vi "Create CE measurements for SS.vi"(8 "error in (no error)":errorcluster, 11 "SS measurement":T2 {"PJVS reference voltages array of vector cluster"."PJVS reference voltages vector" format="%#_3p"; "PJVS frequencies (Hz)" format="%#_3p"; "Record lengths (multiples of periods)" format="%#_3p"; "Sampling frequencies (Hz)" format="%#_3p"; "Signal amplitudes (V)" format="%#_3p"; "Signal frequencies (Hz)" format="%#_3p"}) -> (0 "error out":errorcluster, 1 "CE measurement after":T1={"Signal frequencies (Hz) T"=[1000.0], "Signal amplitudes (V) T"=[0.707], "Sampling frequencies (Hz) T"=[10000000.0], "Record lengths (multiples of periods) T"=[10000.0], "TWM data root directory"=path "", "TWM mreasurements directories"=[], "Calculate RMS from samples"=FALSE, "Algorithm to use"="TWM-WFFT", "Quantity to read"="TWM-WFFT", "Settle down after AC source change (s) T"=1.0, "Skip PJVS setup"=FALSE, "Measurement template file"=path "", "Row of START keyword T"=0, "Row of STOP keyword T"=0, "Measurement template line T"=[], "Switch position T"=[10000.0], "FR fit mat file T"=path "", "Recalculate-skip already calculated"=FALSE} {"Switch position T" format="%#_3p"; "Record lengths (multiples of periods) T" format="%#_3p"; "Sampling frequencies (Hz) T" format="%#_3p"; "Signal amplitudes (V) T" format="%#_3p"; "Signal frequencies (Hz) T" format="%#_3p"}, 2 "CE measurement before":T1={"Signal frequencies (Hz) T"=[1000.0], "Signal amplitudes (V) T"=[0.707], "Sampling frequencies (Hz) T"=[10000000.0], "Record lengths (multiples of periods) T"=[10000.0], "TWM data root directory"=path "", "TWM mreasurements directories"=[], "Calculate RMS from samples"=FALSE, "Algorithm to use"="TWM-WFFT", "Quantity to read"="TWM-WFFT", "Settle down after AC source change (s) T"=1.0, "Skip PJVS setup"=FALSE, "Measurement template file"=path "", "Row of START keyword T"=0, "Row of STOP keyword T"=0, "Measurement template line T"=[], "Switch position T"=[10000.0], "FR fit mat file T"=path "", "Recalculate-skip already calculated"=FALSE} {"Switch position T" format="%#_3p"; "Record lengths (multiples of periods) T" format="%#_3p"; "Sampling frequencies (Hz) T" format="%#_3p"; "Signal amplitudes (V) T" format="%#_3p"; "Signal frequencies (Hz) T" format="%#_3p"}, 3 "SS measurement out":T2={"Signal frequencies (Hz)"=[1000.0], "Signal amplitudes (V)"=[0.707], "Sampling frequencies (Hz)"=[10000000.0], "Record lengths (multiples of periods)"=[10000.0], "Calculate results"=FALSE, "Algorithm"="TWM-PJVSSubS", "TWM data directories"=[], "TWM data directories relative"=[], "Settle down after AC source change (s)"=1.0, "PJVS frequencies (Hz)"=[1000.0], "PJVS reference voltages array of vector cluster"=[], "Requested PJVS steps"=[20], "Measure CE"=FALSE, "Measure CE before"=FALSE, "Measure CE after"=FALSE, "Single point CE measurement"=FALSE, "original CE template path"=path "", "new CE template path before SS"=path "", "new CE template path before SS relative"=path "", "new CE template path after SS"=path "", "new CE template path after SS relative"=path "", "original CE fit path"=path "", "new CE fit path before SS"=path "", "new CE fit path before SS relative"=path "", "new CE fit path after SS"=path "", "new CE fit path after SS relative"=path "", "Measure digitizer gain"=FALSE, "Measure digitizer gain before"=FALSE, "Measure digitizer gain after"=FALSE, "Digitizer gain"=0.0, "Data folder"=path "", "FR fit path"=path "", "new FR fit path relative"=path "", "Rs"=0, "Re"=0, "SS measurement info files"=[]} {"PJVS reference voltages array of vector cluster"."PJVS reference voltages vector" format="%#_3p"; "PJVS frequencies (Hz)" format="%#_3p"; "Record lengths (multiples of periods)" format="%#_3p"; "Sampling frequencies (Hz)" format="%#_3p"; "Signal amplitudes (V)" format="%#_3p"; "Signal frequencies (Hz)" format="%#_3p"})   [LabVIEW 2020]
doc: "Prepare CE measurement for SS measurement - proper paths, if needed modify for single point CE mesurement."
uses:
  SS Measurement/Type definitions/SS measurement.ctl
  CE Measurement/Type definitions/CE measurement.ctl
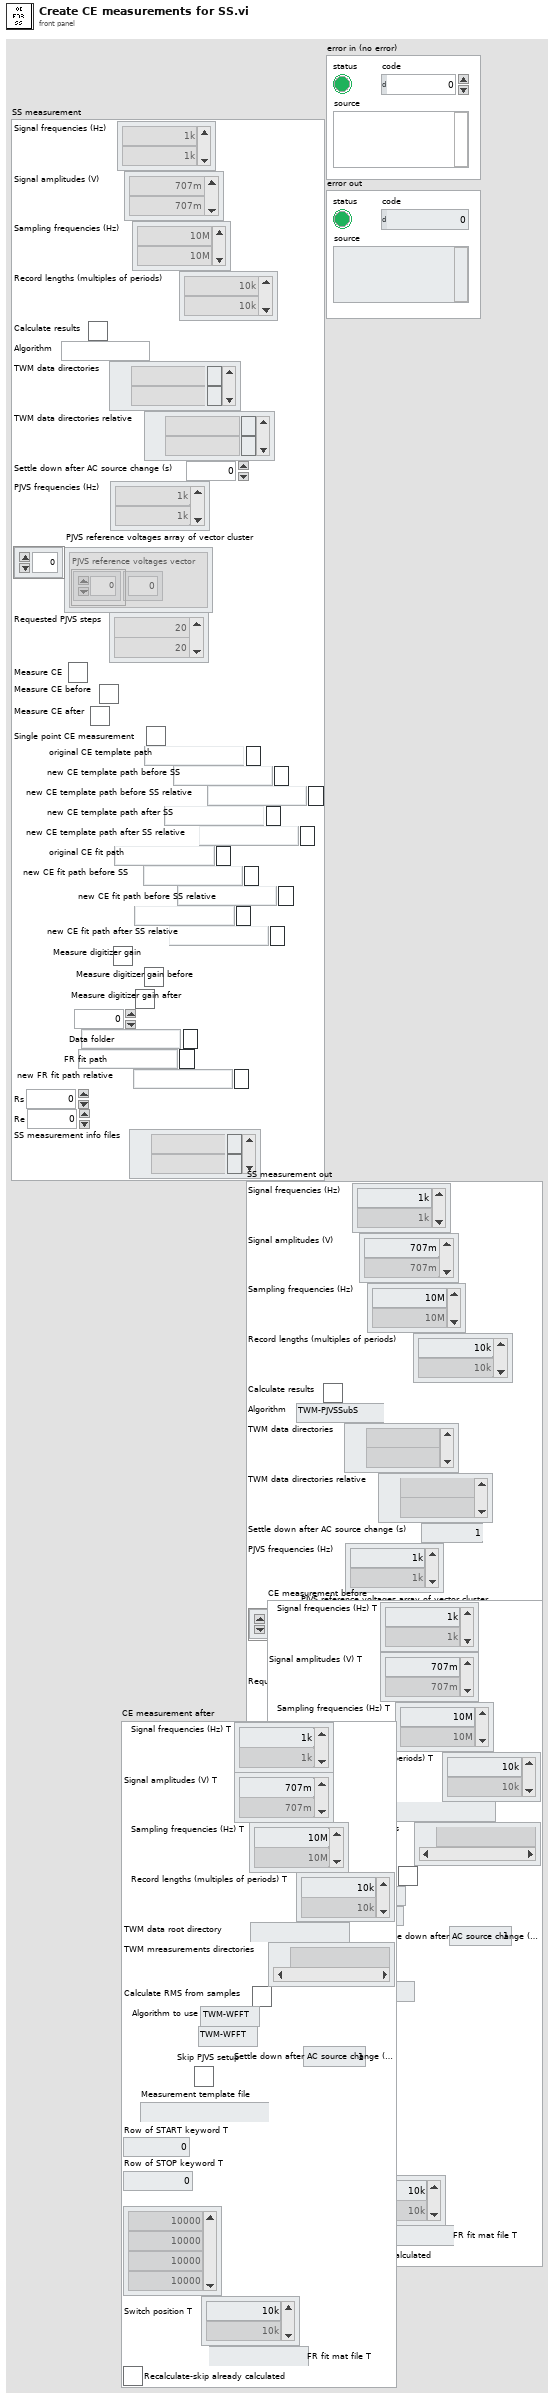
[diagram p1: front panel]
types:
  T1 = typedef "CE measurement.ctl" = cluster{"Signal frequencies (Hz) T":dbl[], "Signal amplitudes (V) T":dbl[], "Sampling frequencies (Hz) T":dbl[], "Record lengths (multiples of periods) T":dbl[], "TWM data root directory":path, "TWM mreasurements directories":path[], "Calculate RMS from samples":bool, "Algorithm to use":string, "Quantity to read":string, "Settle down after AC source change (s) T":dbl, "Skip PJVS setup":bool, "Measurement template file":path, "Row of START keyword T":i32, "Row of STOP keyword T":i32, "Measurement template line T":i32[], "Switch position T":dbl[], "FR fit mat file T":path, "Recalculate-skip already calculated":bool}
  T2 = typedef "SS measurement.ctl" = cluster{"Signal frequencies (Hz)":dbl[], "Signal amplitudes (V)":dbl[], "Sampling frequencies (Hz)":dbl[], "Record lengths (multiples of periods)":dbl[], "Calculate results":bool, "Algorithm":string, "TWM data directories":path[], "TWM data directories relative":path[], "Settle down after AC source change (s)":dbl, "PJVS frequencies (Hz)":dbl[], "PJVS reference voltages array of vector cluster":cluster{"PJVS reference voltages vector":dbl[]}[], "Requested PJVS steps":u32[], "Measure CE":bool, "Measure CE before":bool, "Measure CE after":bool, "Single point CE measurement":bool, "original CE template path":path, "new CE template path before SS":path, "new CE template path before SS relative":path, "new CE template path after SS":path, "new CE template path after SS relative":path, "original CE fit path":path, "new CE fit path before SS":path, "new CE fit path before SS relative":path, "new CE fit path after SS":path, "new CE fit path after SS relative":path, "Measure digitizer gain":bool, "Measure digitizer gain before":bool, "Measure digitizer gain after":bool, "Digitizer gain":dbl, "Data folder":path, "FR fit path":path, "new FR fit path relative":path, "Rs":i32, "Re":i32, "SS measurement info files":path[]}
  T3 = typedef "Type definitions to be saved.ctl" = cluster{"Common properties":T4, "AC Source":T5, "DC meter":T7, "CE measurement":T1, "FR measurement":T9, "FR template":T10, "CE template":T11, "PJVS":T12, "SS measurement":T2, "AC sync source":T5, "DG measurement":T16}
  T4 = typedef "Common properties.ctl" = cluster{"Measurement status ref":refnum<vi>, "TWM Status ref":refnum<vi>, "Abort ref":refnum<vi>, "Skip waiting ref":refnum<vi>, "GNU Octave path":path, "TWM+QWTB path":path, "lvlib path":path, "TWM pipe":string, "PJVS status ref":refnum<vi>, "WAC path":path}
  T5 = typedef "AC Source.ctl" = cluster{"AC Source type":T6, "VISA":refnum<visa-resource-name>, "Ref. clock (Hz)":dbl, "status ref":refnum<vi>, "Fluke 57XX wideband output":bool, "Fluke 57XX ignore errors":bool, "Synchronization by AC signal":bool}
  T6 = typedef "AC Source type.ctl" = enum16{"Fluke 5XXX calibrator", "Tektronix AFG3000 series", "dummy", "Agilent 331xxA to 332xxA", "Agilent 335xxA to 336xxA"}
  T7 = typedef "DC meter.ctl" = cluster{"DC meter type":T8, "DC meter VISA":refnum<visa-resource-name>, "NPLC":dbl, "status ref":refnum<vi>}
  T8 = typedef "DC meter type.ctl" = enum16{"H/A/K 3458", "Fluke 8508A", "dummy", "Keithley 2182"}
  T9 = typedef "FR measuement.ctl" = cluster{"Measurement frequencies (Hz)":dbl[], "Sampling frequency (Hz)":dbl, "Signal amplitude (V)":dbl, "AC-DC settle time (s)":dbl, "Record length (multiples of period)":dbl[], "Measurement template file":path, "Row of START keyword":i32, "Row of STOP keyword":i32, "Calculate RMS from samples":bool, "AC-DC warm up time (s)":dbl, "Measurement template line":i32[], "DC meter readings No.":i32, "Algorithm":string, "Simultaneous measurement":bool, "Recalculate-skip already calculated":bool}
  T10 = typedef "FR template.ctl" = cluster{"Keywords column":i32, "Sig. freq. column":i32, "Rec. len. column":i32, "Meas. points. row min to read":i32, "Meas. points. row max to read":i32, "Properties column":i32, "Properties row start":i32, "Properties row end":i32, "Keyword START regexp":string, "Keyword STOP regexp":string, "HW data column":i32, "HW data row start":i32, "HW data row end":i32, "TIme and date column start":i32, "Digitizer value column start ":i32, "DC mean column start ":i32, "DC readings column start":i32}
  T11 = typedef "CE template.ctl" = cluster{"Keywords column":i32, "Sig. freq. column":i32, "Rec. len. column":i32, "Switch pos column":i32, "Meas. points. row min to read":i32, "Meas. points. row max to read":i32, "Properties column":i32, "Properties row start":i32, "Properties row end":i32, "Keyword START regexp":string, "Keyword STOP regexp":string, "HW data column":i32, "HW data row start":i32, "HW data row end":i32, "TIme and date column start":i32, "Digitizer value column start ":i32}
  T12 = typedef "PJVS.ctl" = cluster{"PJVS type":T13, "Status Refnum":refnum<vi>, "AC-supraVOLTcontrol":cluster{"IP address:port (0.0.0.0:0000)":string, "Timeouts":T14, "Simulation mode":bool, "Debug mode":bool}, "NPL bias source":cluster{"DataSocketCluster":T15}, "Manual PJVS":cluster{"PJVS frequency (Hz)":dbl, "Reference voltages (V)":dbl[], "File with PJVS voltages":path}, "VTT PJVS":cluster{"some VTT only property":string}}
  T13 = typedef "PJVS Type.ctl" = enum16{"AC-supraVOLTcontrol", "JV modified NPL bias control", "Manual PJVS", "VTT PJVS"}
  T14 = typedef "ACSVcontrol-driver.lvlib/Timeouts.ctl" = cluster{"TCP Read & Write (ms)":i32, "Sensors readout":i32, "PJVS setup":i32, "Nullmeter readout":i32, "Multiplexer setup":i32, "57XX setup":i32, "Generator setup":i32, "Synthesizer setup":i32, "Sampler readout":i32}
  T15 = typedef "DataSocketCluster external.ctl" = cluster{"Server Machine":string, "Client Machine":string, "Data":string, "TimeStamp":dbl, "Count":i32, "Target Process":string}
  T16 = typedef "DG measurement.ctl" = cluster{"Sampling frequencies (Hz)":dbl[], "Requested PJVS frequencies (Hz)":dbl[], "Requested PJVS waveform amplitudes (V)":dbl[], "Record lengths (multiples of PJVS periods)":dbl[], "Requested PJVS steps":u32[], "Switch position":dbl, "Settle down after PJVS change (s)":dbl, "Rs":i32, "Re":i32, "Algorithm":string, "Calculate results":bool, "Data folder":path, "TWM data directories":path[], "TWM data directories relative":path[], "DG measurement info files":path[], "Set PJVS frequencies (Hz)":dbl[], "Set PJVS reference voltages array of vector cluster":cluster{"PJVS reference voltages vector":dbl[]}[], "Set PJVS steps":u32[]}
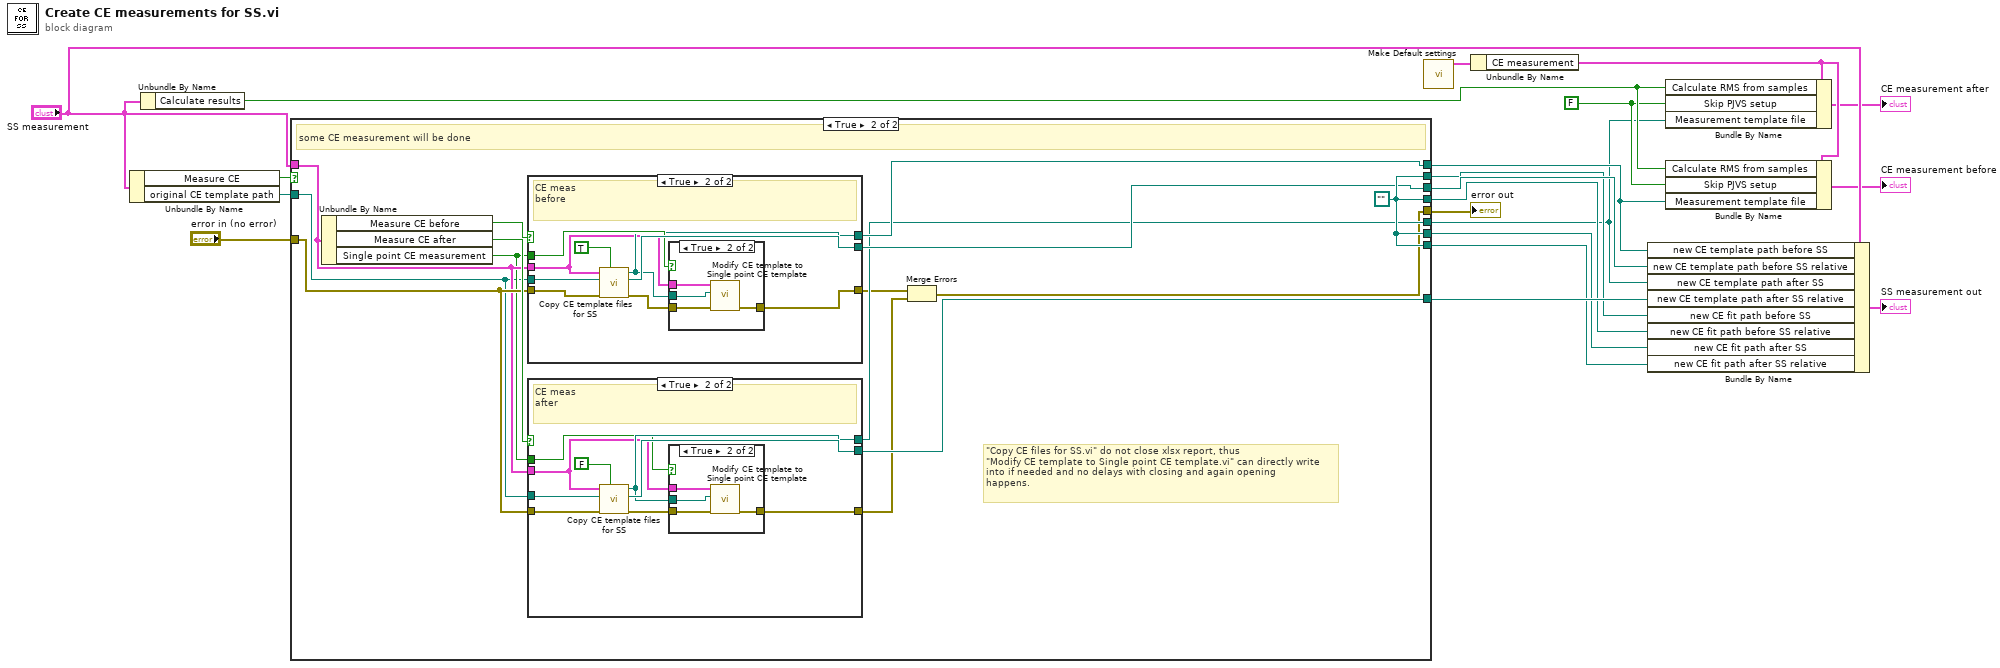
[diagram p0: block diagram]
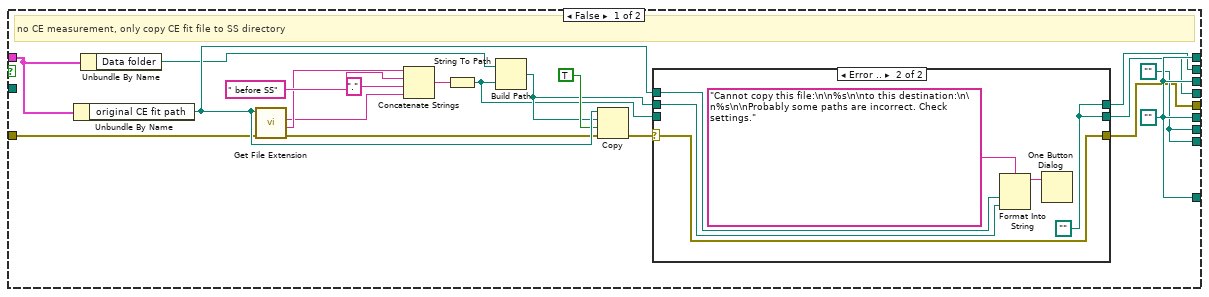
[diagram p2: hidden frame]
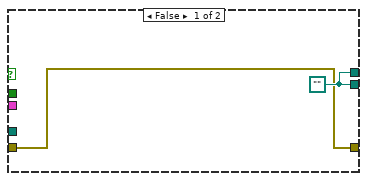
[diagram p4: hidden frame]
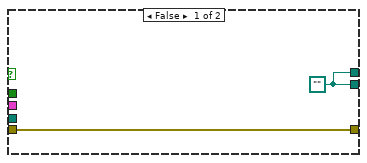
[diagram p6: hidden frame]
diagram:
  w3 = FALSE ("Skip PJVS setup")
  n1 = Unbundle By Name("SS measurement") -> ("Measure CE"=w10:bool, "original CE template path"=w11:path)
  n2 = Unbundle By Name("SS measurement") -> ("Calculate results"=w4:bool)
  n3 = case shown="True" w10 {
    tunnel: [w39 w60] -> w2
    tunnel: [w39 w59] -> w19
    tunnel: [w39 w57] -> w1
    tunnel: [w39 w56] -> w18
    tunnel: "SS measurement" -> [w37 w51]
    tunnel: [w35 w62] -> w17
    tunnel: [w34 w62] -> w16
    tunnel: [w33 w62] -> w15
    tunnel: [w33 w62] -> w14
    tunnel: "error in (no error)" -> [w31 w55]
    tunnel: [w32 w52] -> w12
    tunnel: w11 -> [_ w49]
    frame False {
      w33 = path ""
      w39 = path ""
      # "no CE measurement, only copy CE fit file to SS directory"
      n4 = Unbundle By Name(w37) -> ("original CE fit path"=w36:path)
      n5 = Unbundle By Name(w37) -> ("Data folder"=w21:path)
      n6 = call <vilib>:"Get File Extension.vi"("error in (no error)"=w31, "file"=w36) -> ("error out"=w25:errorcluster, "filename without extension"=w28:string, "lowercase file extension"=w26:string)  [unwired: 5 in, 2 out]
      n7 = Concatenate Strings(w28, " before SS" ("string"), "." ("string"), w26) -> (w29:string)
      n8 = String To Path(string=w29) -> (path=w22:path)
      n9 = Build Path(base path=w21, name or relative path=w22) -> (appended path=w23:path)
      n10 = Copy(8:w25, 9:TRUE ("overwrite (F)"), 10:w23, 11:w36) -> (0:w24:errorcluster)  [unwired: 1 in, 2 out]
      n11 = case shown="Error .." w24 {
        selector: w24 -> [w42 w46]
        tunnel: [w42 w46] -> w32
        tunnel: w36 -> [_ w45]
        tunnel: w23 -> [w41 w44]
        tunnel: [w41 w43] -> w35
        tunnel: [w40 w43] -> w34
        tunnel: w22 -> [w40 _]
        frame No Error {
        }
        frame Error {
          w43 = path ""
          n12 = Format Into String(format string="Cannot copy this file:\n\n%s\n\nto this destination:\n\n%s\n\nProbably some paths are incorrect. Check settings.", w45, w44) -> (resulting string=w47:string)  [unwired: 2 in, 1 out]
          n13 = One Button Dialog(message=w47) -> ()  [unwired: 1 in, 1 out]
        }
      }
    }
    frame True {
      w62 = path ""
      # "\"Copy CE files for SS.vi\" do not close xlsx report, thus \n\"Modify CE template to Single point CE template.vi\" can directly write\ninto if needed and no delays with closing and again opening\nhappens."
      # "some CE measurement will be done"
      n14 = Unbundle By Name(w51) -> ("Measure CE before"=w61:bool, "Measure CE after"=w58:bool, "Single point CE measurement"=w50:bool)
      n15 = case shown="True" w61 {
        tunnel: w51 -> [_ w82]
        tunnel: [w80 w84] -> w60
        tunnel: [w80 w89] -> w59
        tunnel: [w79 w85] -> w54
        tunnel: w55 -> [w79 w88]
        tunnel: w50 -> [_ w87]
        tunnel: w49 -> [_ w83]
        frame False {
          w80 = path ""
        }
        frame True {
          # "CE meas\nbefore"
          n16 = call "Copy CE template files for SS.vi"("before SS? (T)"=TRUE, "error in (no error)"=w88, "CE template file"=w83, "SS measurement"=w82) -> ("error out"=w86:errorcluster, "new CE template file relative"=w89:path, "new CE template file"=w84:path)  [unwired: 4 in, 1 out]
          n17 = case shown="True" w87 {
            tunnel: w86 -> [w90 w94]
            tunnel: [w90 w93] -> w85
            tunnel: w84 -> [_ w91]
            tunnel: w82 -> [_ w92]
            frame False {
            }
            frame True {
              n18 = call "Modify CE template to Single point CE template.vi"("error in (no error)"=w94, "Measurement template file"=w91, "SS measurement"=w92) -> ("error out"=w93:errorcluster)  [unwired: 8 in]
            }
          }
        }
      }
      n19 = case shown="True" w58 {
        tunnel: w51 -> [_ w66]
        tunnel: [w64 w69] -> w57
        tunnel: [w64 w73] -> w56
        tunnel: w55 -> [w63 w72]
        tunnel: [w63 w70] -> w53
        tunnel: w50 -> [_ w68]
        tunnel: w49 -> [_ w67]
        frame False {
          w64 = path ""
        }
        frame True {
          # "CE meas\nafter"
          n20 = call "Copy CE template files for SS.vi"("before SS? (T)"=FALSE, "error in (no error)"=w72, "CE template file"=w67, "SS measurement"=w66) -> ("error out"=w71:errorcluster, "new CE template file relative"=w73:path, "new CE template file"=w69:path)  [unwired: 4 in, 1 out]
          n21 = case shown="True" w68 {
            tunnel: w71 -> [w74 w78]
            tunnel: [w74 w77] -> w70
            tunnel: w69 -> [_ w75]
            tunnel: w66 -> [_ w76]
            frame False {
            }
            frame True {
              n22 = call "Modify CE template to Single point CE template.vi"("error in (no error)"=w78, "Measurement template file"=w75, "SS measurement"=w76) -> ("error out"=w77:errorcluster)  [unwired: 8 in]
            }
          }
        }
      }
      n23 = Merge Errors(w54, w53) -> (w52:errorcluster)
    }
  }
  "error out" <- w12
  n24 = call "Make Default settings.vi"() -> ("TD to be saved"=w9:T3)  [unwired: 11 in]
  n25 = Unbundle By Name(w9) -> ("CE measurement"=w6:T1)
  n26 = Bundle By Name(cluster="SS measurement", "new CE template path before SS"=w2, "new CE template path before SS relative"=w19, "new CE template path after SS"=w1, "new CE template path after SS relative"=w18, "new CE fit path before SS"=w17, "new CE fit path before SS relative"=w16, "new CE fit path after SS"=w15, "new CE fit path after SS relative"=w14) -> (→"SS measurement out":T2)
  n27 = Bundle By Name(cluster=w6, "Calculate RMS from samples"=w4, "Skip PJVS setup"=w3, "Measurement template file"=w1) -> (→"CE measurement after":T1)
  n28 = Bundle By Name(cluster=w6, "Calculate RMS from samples"=w4, "Skip PJVS setup"=w3, "Measurement template file"=w2) -> (→"CE measurement before":T1)
